vi "Get Default Path.vi"(8 "error in (no error)":errorcluster, 10 "VI Refnum":refnum<vi>, 11 "Save Restore Settings in":refnum<class "Save Restore Settings.lvclass">) -> (0 "error out":errorcluster, 2 "Default Path":path, 3 "Save Restore Settings out":refnum<class "Save Restore Settings.lvclass">)   [LabVIEW 2020, in "Save Restore Settings.lvclass"]
uses:
  <userlib>/_MGI/Application Control/MGI Save Restore Settings/Save Restore Settings.lvclass
  <userlib>/_MGI/File/MGI Windows Folder Enum.ctl
  <userlib>/_MGI/File/MGI Create Directory Chain Behavior Enum.ctl
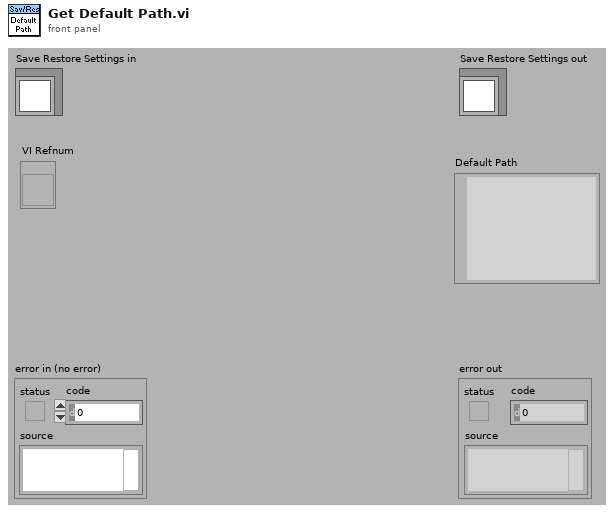
[diagram p1: front panel]
types:
  T1 = typedef "MGI Create Directory Chain Behavior Enum.ctl" = enum16{"Auto Detect", "Path Contains a File", "Path Does Not Contain a File"}
  T2 = typedef "MGI Windows Folder Enum.ctl" = enum32{"Desktop", "Err<Internet>", "Programs", "Err<Controls>", "Err<Printers>", "Personal (MyDocuments)", "Favorites", "Startup", "Recent", "SendTo", "Err<RecycleBin>", "StartMenu", "Err<MyDocuments>", "MyMusic", "MyVideo", "Err<0x000F>", "DesktopDirectory", "Err<Drives>", "Err<Network>", "NetHood", "Fonts", "Templates", "CommonStartMenu", "CommonPrograms", "CommonStartup", "CommonDesktopDirectory", "AppData", "PrintHood", "LocalAppData", "Err<AltStartup>", "Err<CommonAltStartup>", "CommonFavorites", "InternetCache", "Cookies", "History", "CommonAppData", "Windows", "System", "ProgramFiles", "MyPictures", "Profile", "System32", "Err<0x002A>", "ProgramFilesCommon", "Err<0x002C>", "CommonTemplates", "CommonDocuments", "CommonAdminTools", "AdminTools"}
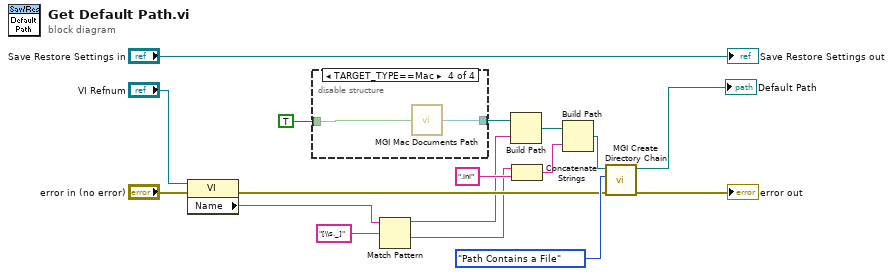
[diagram p0: block diagram]
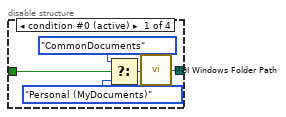
[diagram p2: hidden frame]
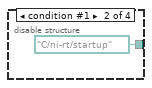
[diagram p3: hidden frame]
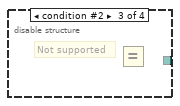
[diagram p4: hidden frame]
diagram:
  n1 = property class="VI"(reference="VI Refnum", error in="error in (no error)") -> (error out=w5:errorcluster, "Name"=w3:string)  [unwired: 1 out]
  n2 = disable-structure shown="TARGET_TYPE==Mac" {
    disable-tunnel: [w22 path "C:/ni-rt/startup" ("Path") _ w24] -> w10
    disable-tunnel: TRUE ("All Users? (True)") -> [w18 _ _ w25]
    frame condition #0 (active) {
      n3 = Select(t=MGI_Windows_Folder_Enum."CommonDocuments" ("Special Folder"), s=w18, f=MGI_Windows_Folder_Enum."Personal (MyDocuments)" ("Special Folder")) -> (s? t:f=w19:T2)
      n4 = call <userlib>:"MGI Windows Folder Path.vi"("Windows Folder"=w19) -> ("Path"=w22:path)
    }
    frame condition #1 {
    }
    frame condition #2 {
      # "Not supported"
      n5 = Equal?() -> ()  [unwired: 2 in, 1 out]
    }
    frame condition #3 {
      n6 = call <userlib>:"MGI Mac Documents Path.vi"("User Documents? (F: Shared Documents)"=w25) -> ("Path"=w24:path)
    }
  }
  n7 = Match Pattern(string=w3, regular expression="[\\s._]") -> (before substring=w2:string, after substring=w1:string)  [unwired: 1 in, 2 out]
  n8 = Build Path(base path=w10, name or relative path=w2) -> (appended path=w13:path)
  n9 = Concatenate Strings(w1, ".ini" ("string")) -> (w12:string)
  n10 = Build Path(base path=w13, name or relative path=w12) -> (appended path=w14:path)
  n11 = call <userlib>:"MGI Create Directory Chain.vi"("Error In"=w5, "File Presence (Auto Detect)"=MGI_Create_Directory_Chain_Behavior_Enum."Path Contains a File", "Path"=w14) -> ("Error Out"=→"error out":errorcluster, "Duplicate Path"=→"Default Path":path)  [unwired: 7 in]
  "Save Restore Settings out" <- "Save Restore Settings in"
